vi "build mag reading from readings.vi"(0 "reading":T2, 7 "magnetometer x locations":dbl[](array[numeric])=[0.0, -22.5, -22.5, 45.0], 9 "magnetometer y locations":dbl[](array[numeric])=[0.0, 38.971, -38.971, 0.0], 11 "magnetometer set working in":bool[](array[boolean])) -> (4 "reading out":T1, 6 "reading completed":bool, 15 "mag set working out":bool[](array[boolean]))   [LabVIEW 2017]
uses:
  typedefs/reading.ctl
  typedefs/readingType.ctl
  typedefs/magnetomter reading set.ctl
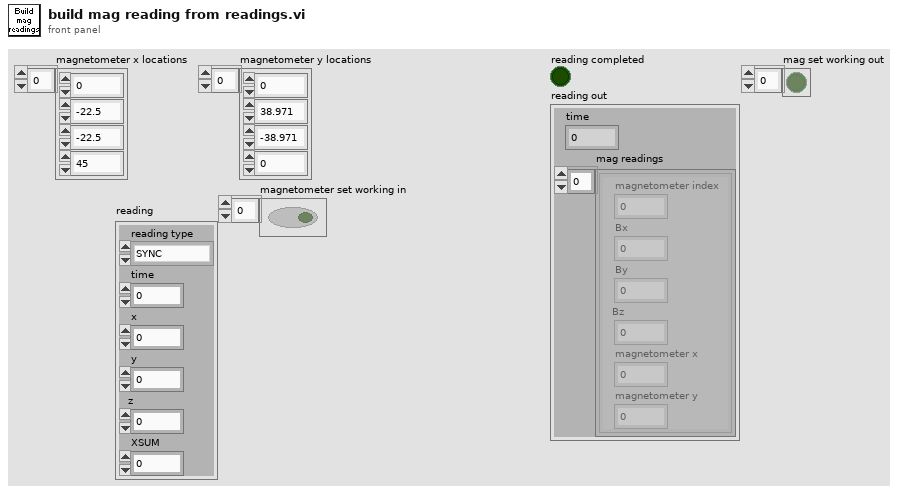
[diagram p1: front panel]
types:
  T1 = typedef "magnetomter reading set.ctl" = cluster{"time":fxp<+,48,48>, "mag readings":cluster{"magnetometer index":dbl, "Bx":dbl, "By":dbl, "Bz":dbl, "magnetometer x":dbl, "magnetometer y":dbl}[]}
  T2 = typedef "reading.ctl" = cluster{"reading type":T3, "time":fxp<+,48,48>, "x":sgl, "y":sgl, "z":sgl, "XSUM":u8}
  T3 = typedef "readingType.ctl" = enum8{"SYNC", "DETVAL", "COILI", "MAGVEC", "ACCVEC", "CROSSING", "MAGVEC0", "MAGVEC1", "MAGVEC2", "MAGVEC3", "MAGVEC4", "MAGVEC5", "MAGVEC6", "MAGVEC7"}
  T4 = cluster{"magnetometer index":dbl, "Bx":dbl, "By":dbl, "Bz":dbl, "magnetometer x":dbl, "magnetometer y":dbl}
  T5 = cluster{"magnetometer index":dbl, "Bx":dbl, "By":dbl, "Bz":dbl, "magnetometer x":dbl, "magnetometer y":dbl}[]
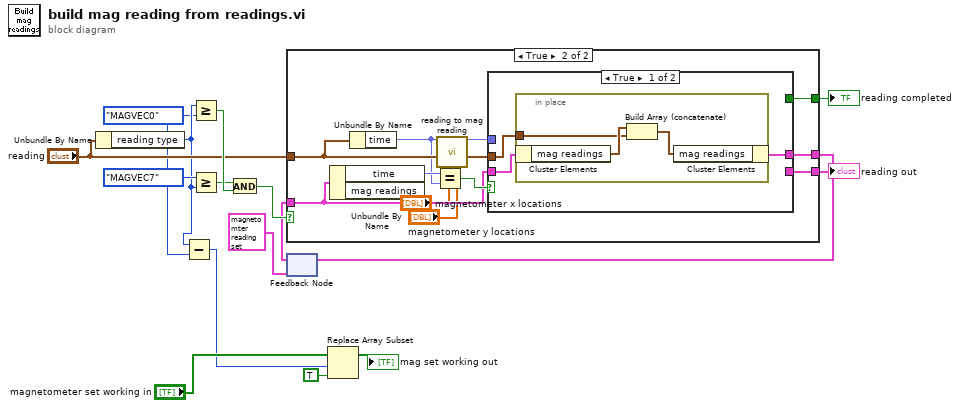
[diagram p0: block diagram]
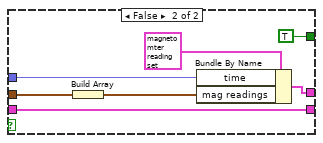
[diagram p3: hidden frame]
diagram:
  w4 = readingType."MAGVEC0" ("y")
  n1 = Unbundle By Name("reading") -> ("reading type"=w5:T3)
  n2 = Subtract(x=w5, y=w4) -> (x-y=w3:u8)
  n3 = Greater Or Equal?(x=w5, y=w4) -> (x >= y?=w16:bool)
  n4 = Greater Or Equal?(x=readingType."MAGVEC7", y=w5) -> (x >= y?=w14:bool)
  n5 = And(x=w14, y=w16) -> (x .and. y?=w13:bool)
  n6 = feedback #1(T1 {"time"=0.0, "mag readings"=[]} ("Magnetometer reading set")) -> (w10:T1)
  n7 = case shown="True" w13 {
    tunnel: "reading" -> [_ w25]
    tunnel: w10 -> [w17 w26]
    tunnel: [w17 w23] -> w9
    tunnel: [_ w22] -> w7
    tunnel: [_ w20] -> w8
    frame False {
    }
    frame True {
      n8 = Unbundle By Name(w26) -> ("time"=w28:fxp<+,48,48>)  [unwired: 1 out]
      n9 = Unbundle By Name(w25) -> ("time"=w21:fxp<+,48,48>)
      n10 = Equal?(x=w28, y=w21) -> (x = y?=w27:bool)
      n11 = call "reading to mag reading.vi"("magnetometer y locations"="magnetometer y locations", "magnetometer x locations"="magnetometer x locations", "reading"=w25) -> ("mag reading"=w24:T4)  [unwired: 8 in]
      n12 = case shown="True" w27 {
        tunnel: w26 -> [w31 w41]
        tunnel: w24 -> [w30 w38]
        tunnel: [w29 w36] -> w23
        tunnel: [_ w41] -> w22
        tunnel: w21 -> [_ w39]
        tunnel: [_ TRUE] -> w20
        frame True {
          n13 = in-place {
            in-place-border: w30 -> [w33]
            n14 = in-place-cluster #2(w31) -> ("mag readings"=w34:T5)
            n15 = Build Array (concatenate)(w34, w33) -> (w32:T5)
            n16 = in-place-cluster #2("mag readings"=w32) -> (w29:T1)
          }
        }
        frame False {
          n17 = Build Array(w38) -> (w37:T5)
          n18 = Bundle By Name(cluster=T1 {"time"=0.0, "mag readings"=[]} ("Magnetometer reading set"), "time"=w39, "mag readings"=w37) -> (w36:T1)
        }
      }
    }
  }
  "reading completed" <- w8
  "reading out" <- w7
  n19 = feedback-in #1(w9) -> ()
  n20 = Replace Array Subset(array="magnetometer set working in", new element=TRUE ("new element/subarray"), index=w3) -> (→"mag set working out":bool[])
